vi "transfer bindings.vi"(8 "error in (no error)":errorcluster, 10 "para1":dbl, 11 "para0":dbl) -> (0 "error out":errorcluster, 1 "function return":i32, 2 "para1 out":dbl, 3 "para0 out":dbl)   [LabVIEW 2020, in "sqlite3.lvlib"]
uses:
  sqlite3.lvlib
  errstr.vi
  bin/sqlite3_64.dll
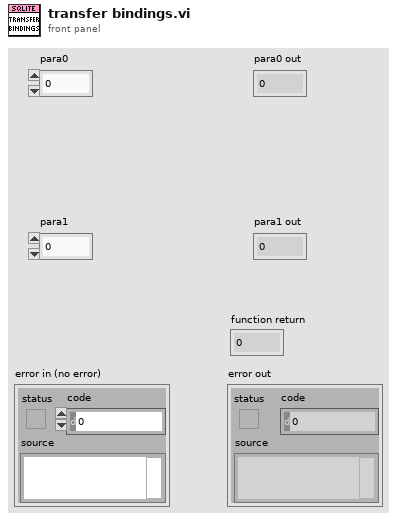
[diagram p1: front panel]
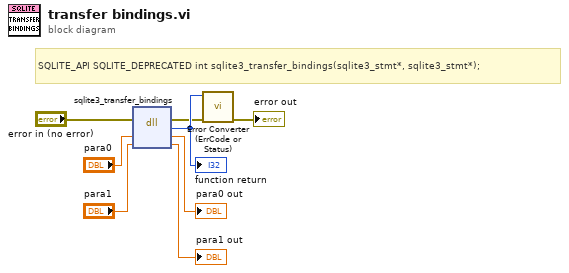
[diagram p0: block diagram]
diagram:
  # "SQLITE_API SQLITE_DEPRECATED int sqlite3_transfer_bindings(sqlite3_stmt*, sqlite3_stmt*);"
  n1 = dll-call lib="C:/Users/Fred.Guo/Desktop/Database-configuration/externals/sqlite3/Source/bin/sqlite3_*.*" fn="sqlite3_transfer_bindings"(error in="error in (no error)", "para0"="para0", "para1"="para1") -> (error out=w2:errorcluster, w8:i32, "para0"=→"para0 out":dbl, "para1"=→"para1 out":dbl)  [unwired: 2 in, 1 out]
  "function return" <- w8
  n2 = call "Error Converter (ErrCode or Status).vi"("error in (no error)"=w2, "error code"=w8) -> ("error out"=→"error out":errorcluster)  [unwired: 9 in]
